vi "DrawBlackKey.vi"(4 "起始音":T1={"音名"=enum."A", "度"=enum."0", "變音記號"=enum.""}, 5 "BlackKeySize":cluster{"Width":i32, "Hieght":i32}={"Width"=10, "Hieght"=97}, 6 "KeyNumber":i32=52, 7 "WhiteKeySize":cluster{"Width":i32, "Hieght":i32}={"Width"=21, "Hieght"=147}, 8 "error in (no error)":errorcluster, 10 "BlackKeyData array":u32[][](array[numeric]), 11 "Image In":T2) -> (0 "error out":errorcluster, 3 "Image Out":T2)   [LabVIEW 2015]
uses:
  <vilib>/vision/Image Controls.llb/IMAQ Image.ctl
  Note.ctl
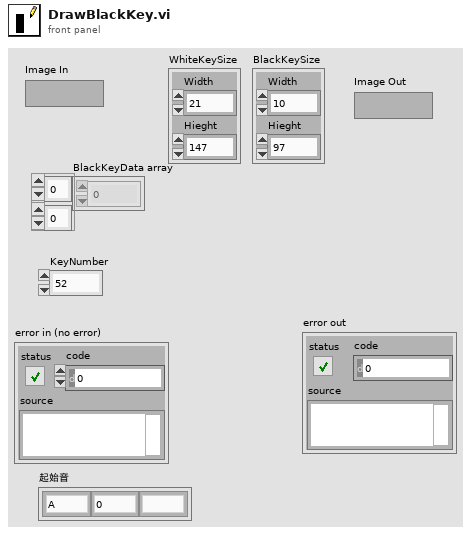
[diagram p1: front panel]
types:
  T1 = typedef "Note.ctl" = cluster{"音名":enum16{"C", "D", "E", "F", "G", "A", "B"}, "度":enum16{"0", "1", "2", "3", "4", "5", "6", "7", "8"}, "變音記號":enum16{"bb", "b", "", "#", "x"}}
  T2 = typedef "IMAQ Image.ctl" = refnum<image>
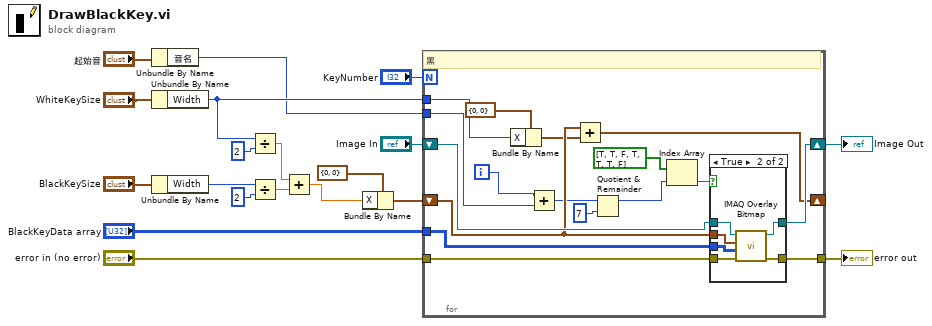
[diagram p0: block diagram]
diagram:
  n1 = Unbundle By Name("起始音") -> ("音名"=w1:enum16{"C", "D", "E", "F", "G", "A", "B"})
  n2 = Unbundle By Name("WhiteKeySize") -> ("Width"=w5:i32)
  n3 = Unbundle By Name("BlackKeySize") -> ("Width"=w3:i32)
  n4 = Divide(x=w5, y=2) -> (x/y=w15:dbl)
  n5 = Divide(x=w3, y=2) -> (x/y=w14:dbl)
  n6 = Add(x=w15, y=w14) -> (x+y=w13:dbl)
  n7 = Bundle By Name(cluster=cluster{"X":i32, "Y":i32} {"X"=0, "Y"=0} ("Top Left Point"), "X"=w13) -> (w17:cluster{"X":i32, "Y":i32})
  n8 = for {
    N: "KeyNumber" -> [_]
    tunnel: "BlackKeyData array" -> [w34]
    shift-right: [w35] -> w11
    shift-left: "Image In" -> [w36]
    shift-right: [w32] -> _
    shift-left: w17 -> [w33]
    tunnel: w5 -> [w28]
    tunnel: "error in (no error)" -> [w29]
    tunnel: [w27] -> w10
    tunnel: w1 -> [w22]
    i -> [w20]
    # "黑"
    n9 = Bundle By Name(cluster=cluster{"X":i32, "Y":i32} {"X"=0, "Y"=0} ("y"), "X"=w28) -> (w30:cluster{"X":i32, "Y":i32})
    n10 = Add(x=w20, y=w22) -> (x+y=w23:i32)
    n11 = Add(x=w33, y=w30) -> (x+y=w32:cluster{"X":i32, "Y":i32})
    n12 = Quotient & Remainder(x=w23, y=7) -> (x-y*floor(x/y)=w21:i32)  [unwired: 1 out]
    n13 = Index Array(array=bool[] [TRUE, TRUE, FALSE, TRUE, TRUE, TRUE, FALSE], index=w21) -> (element=w24:bool)
    n14 = case shown="True" w24 {
      tunnel: w36 -> [w38 w44]
      tunnel: [w38 w43] -> w35
      tunnel: w34 -> [_ w42]
      tunnel: w33 -> [_ w41]
      tunnel: w29 -> [w37 w40]
      tunnel: [w37 w39] -> w27
      frame False {
      }
      frame True {
        n15 = call "IMAQ Overlay Bitmap"("error in (no error)"=w40, "Bitmap"=w42, "Top Left Point"=w41, "Image"=w44) -> ("error out"=w39:errorcluster, "Image Out"=w43:T2)  [unwired: 6 in]
      }
    }
  }
  "Image Out" <- w11
  "error out" <- w10
